vi "Get Results Codes.vi"(0 "ICM Ref In":refnum<class "Modbus Master.lvclass">, 11 "error in (no error)":errorcluster) -> (4 "ICM Ref Out":refnum<class "Modbus Master.lvclass">, 6 ">=4 µ":dbl, 8 ">=6 µ":dbl, 10 ">=14 µ":dbl, 15 "error out":errorcluster)   [LabVIEW 2024]
uses:
  <vilib>/NI/Modbus Library/API/Master/Modbus Master.lvclass
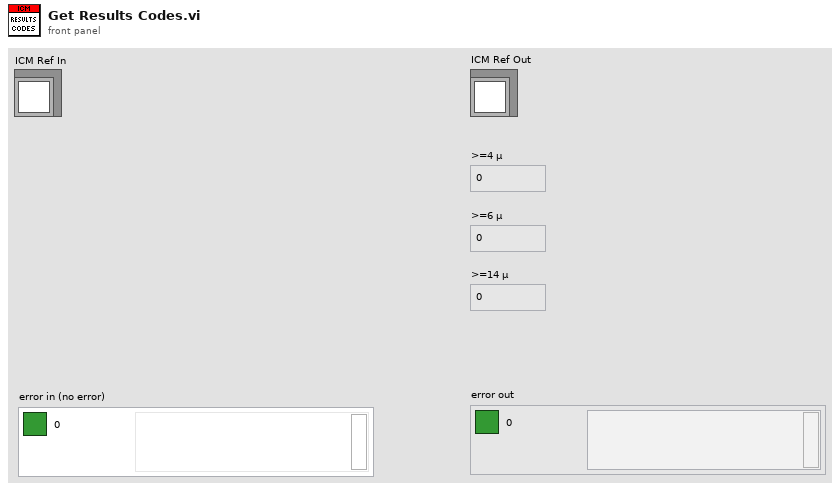
[diagram p1: front panel]
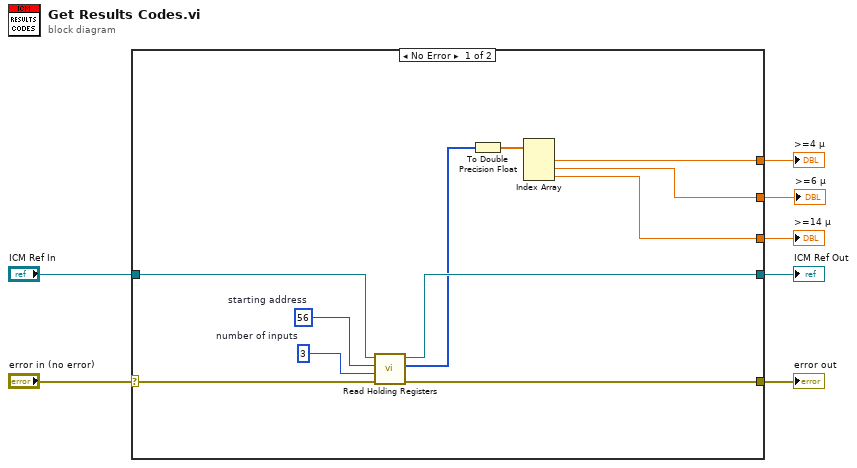
[diagram p0: block diagram]
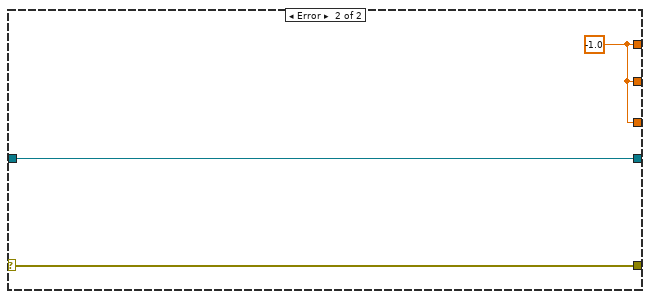
[diagram p2: hidden frame]
diagram:
  n1 = case shown="No Error" "error in (no error)" {
    selector: "error in (no error)" -> [w18 w20]
    tunnel: [w17 w20] -> w7
    tunnel: "ICM Ref In" -> [w16 w21]
    tunnel: [w13 w21] -> w4
    tunnel: [w10 w19] -> w3
    tunnel: [w9 w19] -> w2
    tunnel: [w8 w19] -> w1
    frame No Error {
      w14 = u16 3  # number of inputs
      w15 = u16 56  # starting address
      n2 = call-dynamic "Read Holding Registers.vi"("error in"=w18, "number of inputs"=w14, "starting address"=w15, "Modbus master in"=w16) -> ("error out"=w17:errorcluster, "register values"=w12:u16[], "Modbus master out"=w13:refnum<class "Modbus Master.lvclass">)  [unwired: 5 in]
      n3 = To Double Precision Float(number=w12) -> (double precision float=w11:dbl[])
      n4 = Index Array(array=w11) -> (element #1=w10:dbl, element #2=w9:dbl, element #3=w8:dbl)  [unwired: 3 in]
    }
    frame Error {
      w19 = -1.0
    }
  }
  "error out" <- w7
  "ICM Ref Out" <- w4
  ">=4 µ" <- w3
  ">=6 µ" <- w2
  ">=14 µ" <- w1
